vi "util.convert.u64.to.str.vi"(10 "Final.State":u64[](array[numeric]), 11 "Numeric":i32) -> (3 "String":string)   [LabVIEW 2021]
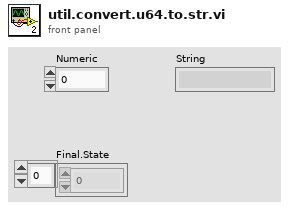
[diagram p1: front panel]
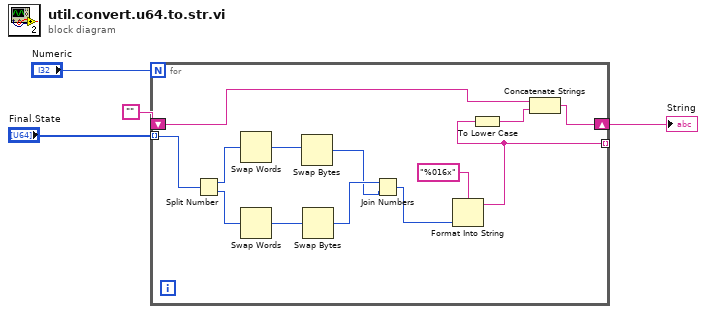
[diagram p0: block diagram]
diagram:
  n1 = for {
    N: "Numeric" -> [_]
    tunnel: "Final.State" -> [w17] mode=indexing
    tunnel: [w5] -> _ mode=indexing
    shift-right: [w10] -> w4
    shift-left: "" -> [w9]
    n2 = Split Number(x=w17) -> (hi(x)=w16:u32, lo(x)=w15:u32)
    n3 = Swap Words(1:w16) -> (0:w14:u32)
    n4 = Swap Words(1:w15) -> (0:w13:u32)
    n5 = Swap Bytes(anything=w14) -> (byte swapped=w11:u32)
    n6 = Swap Bytes(anything=w13) -> (byte swapped=w12:u32)
    n7 = Join Numbers(hi=w12, lo=w11) -> ((hi.lo)=w7:u64)
    n8 = Format Into String(format string="%016x", w7) -> (resulting string=w5:string)  [unwired: 2 in, 1 out]
    n9 = To Lower Case(string=w5) -> (all lower case string=w8:string)
    n10 = Concatenate Strings(w9, w8) -> (w10:string)
  }
  "String" <- w4
